vi "Catapult tester.vi"() -> ()   [LabVIEW 2013]
uses:
  cataplut states.ctl
panel:
  in  "Enum":T1
  in  "Trigger":bool
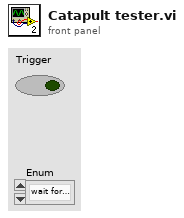
[diagram p1: front panel]
types:
  T1 = typedef "cataplut states.ctl" = enum16{"wait for trigger", "firing", "wench back"}
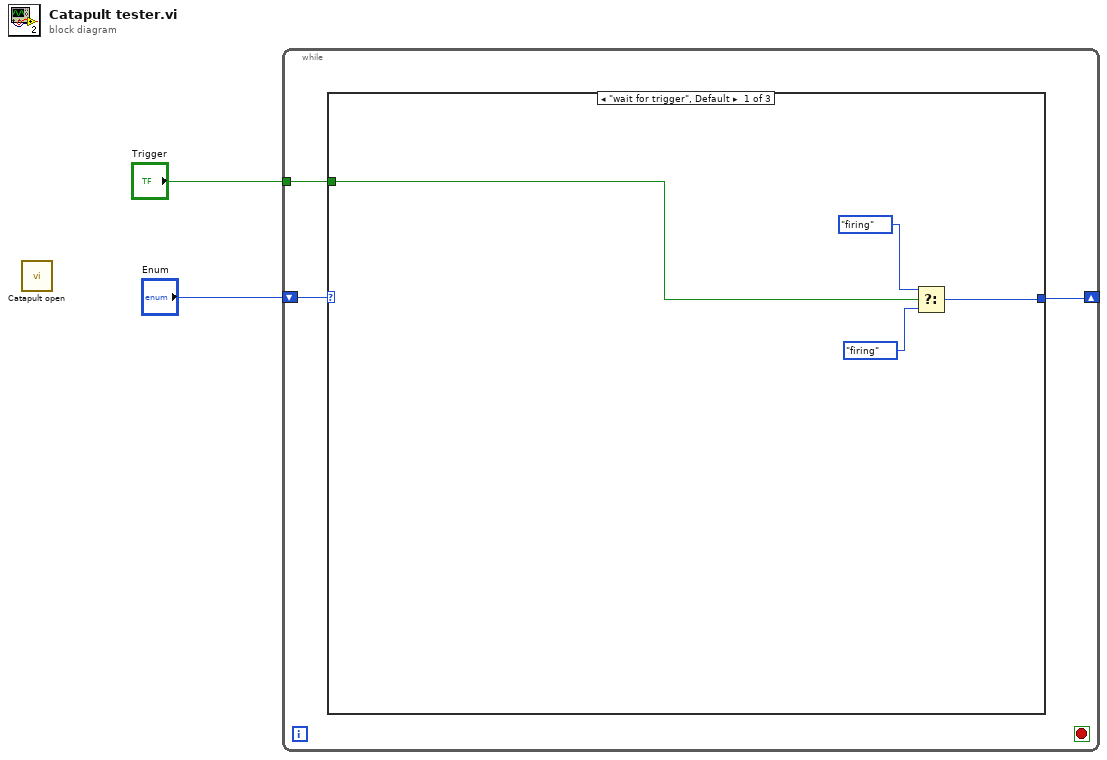
[diagram p0: block diagram]
diagram:
  n1 = call "Catapult open.vi"() -> ()  [unwired: 10 in, 2 out]
  n2 = while {
    shift-right: [w3] -> _
    shift-left: "Enum" -> [w5]
    tunnel: "Trigger" -> [w4]
    stop <- _ stop-if-true
    n3 = case shown="\"wait for trigger\", Default" w5 {
      tunnel: w4 -> [w9 _ _]
      tunnel: [w7 _ _] -> w3
      frame "wait for trigger", Default {
        n4 = Select(t=cataplut_states."firing" ("Enum 2"), s=w9, f=cataplut_states."firing" ("Enum 2")) -> (s? t:f=w7:T1)
      }
      frame "firing" {
      }
      frame "wench back" {
      }
    }
  }
